vi "Update PF Indicator.vi"(6 "PFLabel":refnum<vi>, 8 "Wait? (f)":bool, 9 "Pass? (f)":bool, 11 "error in (no error)":errorcluster) -> (1 "Status Text":string, 3 "error out":errorcluster)   [LabVIEW 2011]
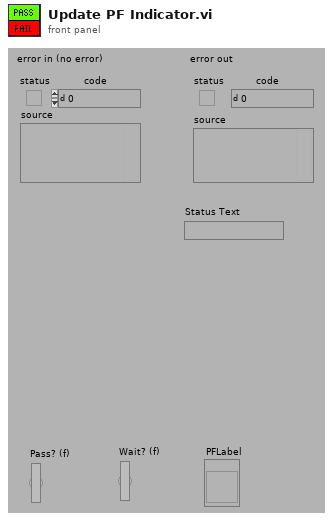
[diagram p1: front panel]
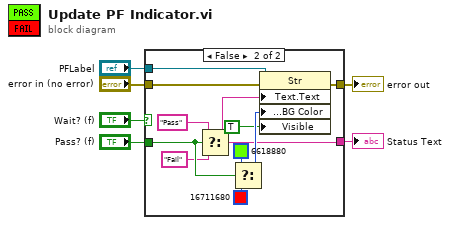
[diagram p0: block diagram]
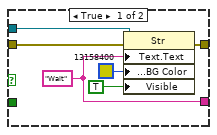
[diagram p2: hidden frame]
diagram:
  n1 = case shown="False" "Wait? (f)" {
    tunnel: "error in (no error)" -> [w12 w23]
    tunnel: "PFLabel" -> [w11 w22]
    tunnel: [w9 w17] -> w4
    tunnel: "Pass? (f)" -> [_ w16]
    tunnel: [w7 w13] -> w1
    frame True {
      w7 = "Wait"
      n2 = property class="Str"(reference=w11, error in=w12, "Text.Text"=w7, "Text.Text Colors:BG Color"=u32 13158400, "Visible"=TRUE) -> (error out=w9:errorcluster)  [unwired: 1 out]
    }
    frame False {
      n3 = Select(t="Pass", s=w16, f="Fail") -> (s? t:f=w13:string)
      n4 = Select(t=u32 6618880, s=w16, f=u32 16711680) -> (s? t:f=w19:u32)
      n5 = property class="Str"(reference=w22, error in=w23, "Text.Text"=w13, "Text.Text Colors:BG Color"=w19, "Visible"=TRUE) -> (error out=w17:errorcluster)  [unwired: 1 out]
    }
  }
  "error out" <- w4
  "Status Text" <- w1
